vi "Read Available Memory.vi"(4 "error in (no error)":errorcluster, 7 "VISA resource name":refnum<visa-resource-name>) -> (0 "error out":errorcluster, 3 "VISA resource name out":refnum<visa-resource-name>)   [LabVIEW 2010, in "Newport ESP301.lvlib"]
doc: "This command reports the amount of unused program memory. The controller has 61440 bytes of non-volatile memory available for permanently storing programs. This command reports the amount not used.\nNote:\nAvailable memory space is updated only after the stored program memory is purged using XX (delete a stored program)s command."
uses:
  <userlib>/Newport ESP301/Newport ESP301.lvlib
panel:
  out "Available Storage Space":i32
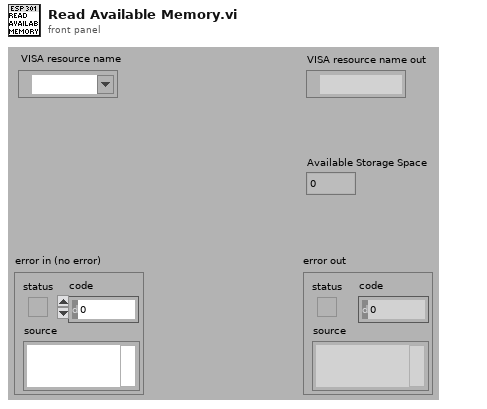
[diagram p1: front panel]
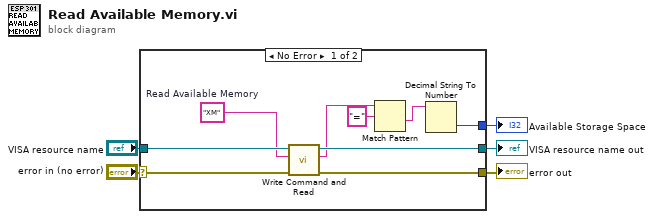
[diagram p0: block diagram]
diagram:
  n1 = case shown="No Error" "error in (no error)" {
    selector: "error in (no error)" -> [w13 w16]
    tunnel: [w11 w16] -> w4
    tunnel: "VISA resource name" -> [w14 w15]
    tunnel: [w12 w15] -> w2
    tunnel: [w10 _] -> w1
    frame No Error {
      w9 = "XM"  # Read Available Memory
      n2 = call <userlib>:"Write Command and Read.vi"("error in (no error)"=w13, "Command"=w9, "VISA resource name"=w14) -> ("error out"=w11:errorcluster, "Returned string"=w8:string, "VISA resource name out"=w12:refnum<visa-resource-name>)  [unwired: 4 in]
      n3 = Match Pattern(string=w8, regular expression="=" ("expression régulière")) -> (after substring=w6:string)  [unwired: 1 in, 3 out]
      n4 = Decimal String To Number(string=w6) -> (number=w10:i32)  [unwired: 2 in, 1 out]
    }
    frame Error {
    }
  }
  "error out" <- w4
  "VISA resource name out" <- w2
  "Available Storage Space" <- w1
